vi "字符串公式求值.vi"() -> ()   [LabVIEW 2022 SP3]
doc: "本VI是为《我和LabVIEW》一书编写的示例。\n关于本书的介绍请参考网页：\nhttp://ruanqizhen.spaces.live.com/blog/cns!5852D4F797C53FB6!4310.entry"
uses:
  <vilib>/gmath/NI_Gmath.lvlib
panel:
  out "公式运算结果":dbl format="%.2f"
  in  "公式":string="sin(pi(1/2)) + 3*5 - 2"
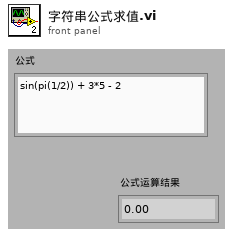
[diagram p1: front panel]
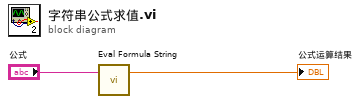
[diagram p0: block diagram]
diagram:
  n1 = call <vilib>:"Eval Formula String.vi"("formula"="公式") -> ("y value"=→"公式运算结果":dbl)  [unwired: 1 in, 1 out]
